vi "9.3. обработка параметров натекания.vi"(11 "param_out":dbl[](array[numeric])) -> (0 "V liter":string, 1 "time":string, 2 "Presure 2":string, 3 "presure 1":string)   [LabVIEW 2016, in "Library.lvlib"]
uses:
  Granule-2000AT/PC/Library.lvlib
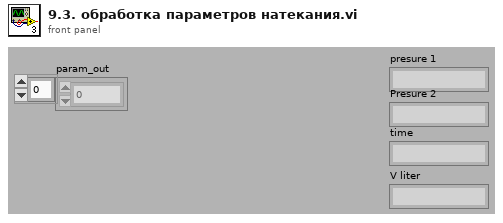
[diagram p1: front panel]
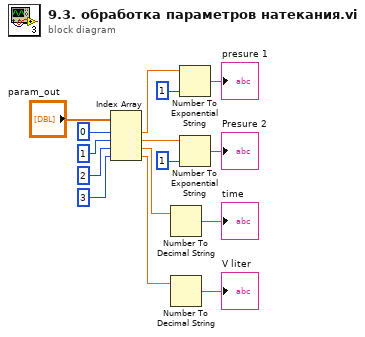
[diagram p0: block diagram]
diagram:
  n1 = Index Array(array="param_out", index #1=0 ("index"), index #2=1 ("index"), index #3=2 ("index"), index #4=3 ("index")) -> (element #1=w10:dbl, element #2=w7:dbl, element #3=w11:dbl, element #4=w2:dbl)
  n2 = Number To Decimal String(number=w11) -> (decimal integer string=→"time":string)  [unwired: 1 in]
  n3 = Number To Decimal String(number=w2) -> (decimal integer string=→"V liter":string)  [unwired: 1 in]
  n4 = Number To Exponential String(number=w10, precision (6)=i16 1) -> (E-format string=→"presure 1":string)  [unwired: 2 in]
  n5 = Number To Exponential String(number=w7, precision (6)=i16 1) -> (E-format string=→"Presure 2":string)  [unwired: 2 in]
